vi "Get as Text.vi"(8 "error in (no error)":errorcluster, 10 "Name Array":string[](array[string]), 11 "JSON Scalar in":refnum<class "JSON Value.lvclass">) -> (0 "error out":errorcluster, 2 "LabVIEW Text":string, 3 "JSON Scalar out":refnum<class "JSON Value.lvclass">)   [LabVIEW 2011, in "JSON Scalar.lvclass"]
doc: "Converts a <b>JSON Value</b> into <b>LabVIEW Text</b>.\nRemoves quotes and escape characters.\n\nCopyright 2012 James David Powell, Shaun Rumbell and Ton Plomp\nMore information on http://lavag.org/topic/16217-cr-json-labview"
uses:
  JSON Scalar.lvclass
  JSON Value/JSON Value.lvclass
panel:
  # "Value formated as LabVIEW text:\n-- no quotes on JSON strings\n-- LabVIEW text encoding <ToDo>\n-- no escaped characters <ToDo>"
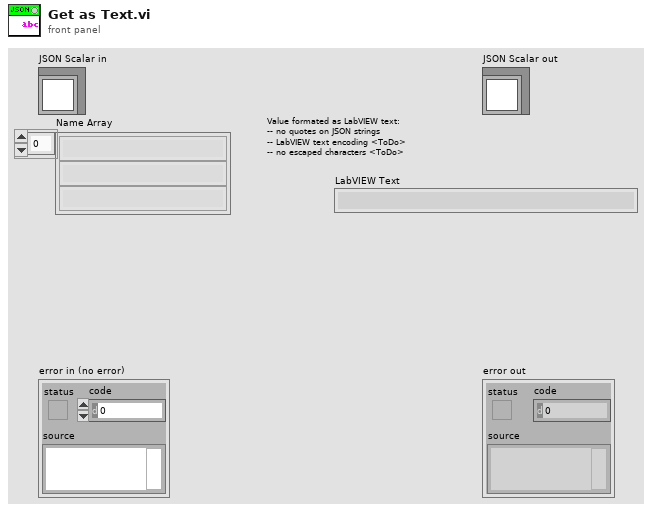
[diagram p1: front panel]
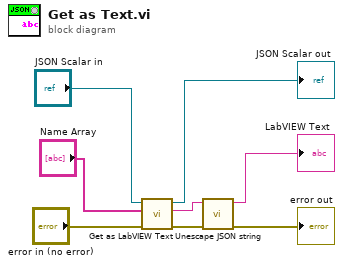
[diagram p0: block diagram]
diagram:
  n1 = call-dynamic "Get as LabVIEW Text.vi"("error in (no error)"="error in (no error)", "Name Array"="Name Array", "JSON Value In"="JSON Scalar in") -> ("error out"=w3:errorcluster, "LabVIEW Text"=w5:string, "JSON Value Out"=→"JSON Scalar out":refnum<class "JSON Value.lvclass">)  [unwired: 6 in]
  n2 = call "Unescape JSON string.vi"("error in (no error)"=w3, "Text (with JSON escapes)"=w5) -> ("error out"=→"error out":errorcluster, "Text (unescaped)"=→"LabVIEW Text":string)  [unwired: 8 in]
